vi "SEQ Obtain.vi"(8 "error in":errorcluster) -> (0 "error out":errorcluster, 3 "queue out":refnum<queue>)   [LabVIEW 2019, in "Initialize.lvlib"]
uses:
  Initialize.lvlib
  SEQ Data.ctl
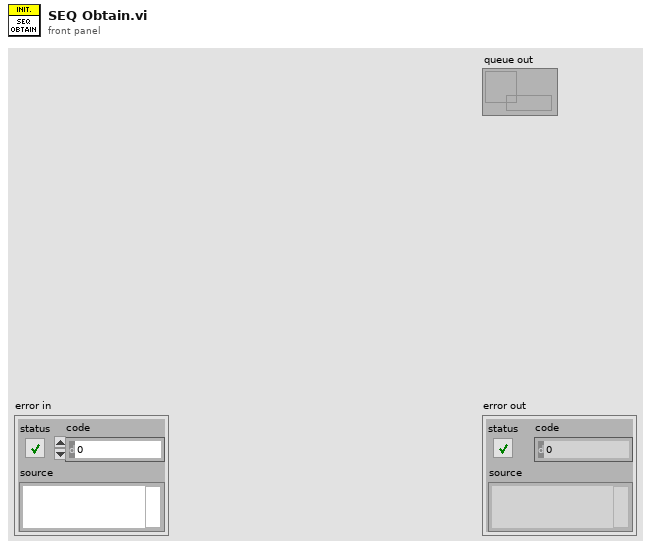
[diagram p1: front panel]
types:
  T1 = typedef "Initialize.lvlib/SEQ Data.ctl" = cluster{"Folder Path":path}
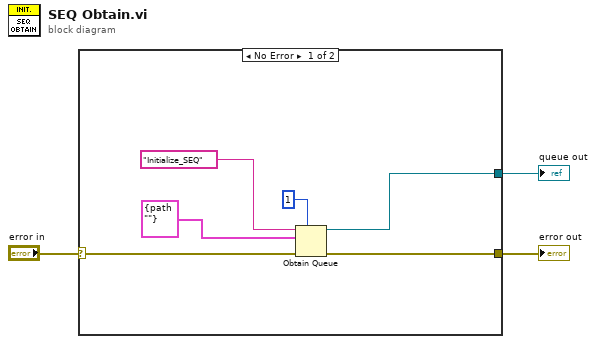
[diagram p0: block diagram]
diagram:
  n1 = case shown="No Error" "error in" {
    selector: "error in" -> [w9 w10]
    tunnel: [w8 w10] -> w2
    tunnel: [w4 _] -> w1
    frame No Error {
      n2 = Obtain Queue(max queue size (-1, unlimited)=1, name (unnamed)="Initialize_SEQ", element data type=T1 {"Folder Path"=path ""} ("Cluster"), error in (no error)=w9) -> (queue out=w4:refnum<queue>, error out=w8:errorcluster)  [unwired: 1 in, 1 out]
    }
    frame Error {
    }
  }
  "error out" <- w2
  "queue out" <- w1
